vi "SavaMeasurement.vi"(0 "error out":errorcluster, 2 "Measurement":string, 4 "refnum out":refnum<file>, 5 "DiodeTemperature":dbl) -> (1 "error out 2":errorcluster, 3 "refnum out 2":refnum<file>)   [LabVIEW 2009]
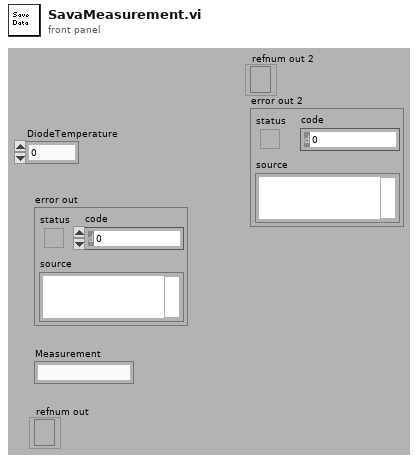
[diagram p1: front panel]
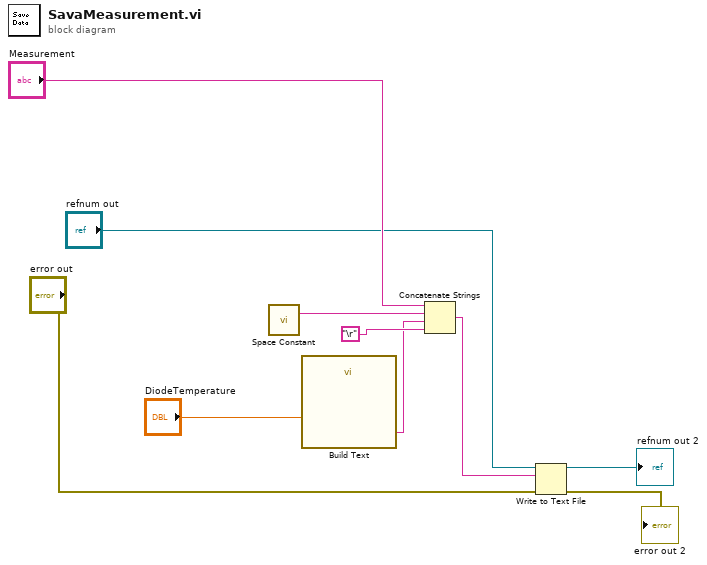
[diagram p0: block diagram]
diagram:
  n1 = call <vilib>:"Space Constant.vi"() -> ("String"=w6:string)
  n2 = call "Build Text"("DiodeTemperature"="DiodeTemperature") -> ("Result"=w7:string)  [unwired: 13 in, 1 out]
  n3 = Concatenate Strings("Measurement", w6, w7, "\r") -> (w9:string)
  n4 = Write to Text File(file (use dialog)="refnum out", text=w9, error in="error out") -> (refnum out=→"refnum out 2":refnum<file>, error out=→"error out 2":errorcluster)  [unwired: 1 in, 1 out]
